vi "Programming Mode.vi"(8 "error in (no error)":errorcluster, 11 "serverName In":string="10.0.18.244") -> (0 "error out":errorcluster, 1 "Programming Mode Out":T1[](array[typedef]), 2 "Cancelled":bool, 3 "serverName Out":string="10.0.18.244")   [LabVIEW 2019, in "SEECD System Explorer.lvlib"]
doc: "This VI detects whether or not target local chassis supports \"Slot Programming Mode\" property.\nIf the case, populated slots have current value for the property displayed and user can change property.\nIf not the case, front-panel is not opened."
uses:
  SEECD System Explorer.lvlib
  Type Defs/Slot - Configuration.ctl
  Type Defs/Slot Programming Mode.ctl
  <vilib>/nisyscfg/Close (Resources).vi
  <vilib>/nisyscfg/Close (Filter).vi
  <vilib>/nisyscfg/Close (System).vi
  <vilib>/nisyscfg/nisyscfg.lvlib
panel:
  in  "Slot 7":T2 caption="Slot"
  in  "Slot 6":T2 caption="Slot"
  in  "Slot 5":T2 caption="Slot"
  in  "Slot 4":T2 caption="Slot"
  in  "Slot 3":T2 caption="Slot"
  in  "Slot 2":T2 caption="Slot"
  in  "Slot 1":T2 caption="Slot"
  in  "Slot 0":T2 caption="Slot"
  in  "User Name":string
  in  "Password":string
  in  "Set all modules to \"Scan Engine\" mode":bool
  in  "Cancel":bool
  in  "OK":bool
  # "Select a programming mode for detected modules and click \"OK\" button."
  # "New\nProgramming Mode"
  # "Current\nProgramming Mode"
  # "Module Name"
  # "Modules Name"
  # "Slot"
  # "Programming Mode"
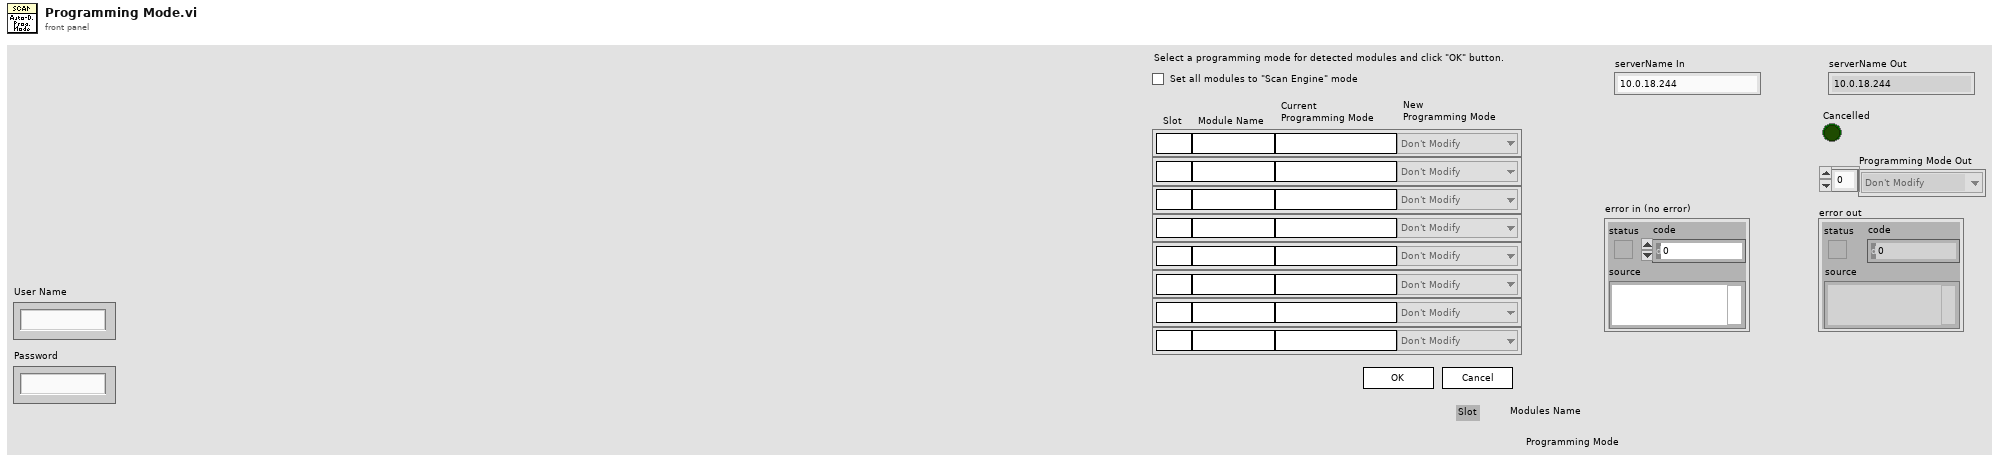
[diagram p1: front panel]
types:
  T1 = typedef "SEECD System Explorer.lvlib/Slot Programming Mode.ctl" = enum16{"Don't Modify", "Scan Engine", "LabVIEW FPGA", "NI-DAQmx"}
  T2 = typedef "SEECD System Explorer.lvlib/Slot - Configuration.ctl" = cluster{"Slot":string, "Module Name":string, "Current Prog Mode":string, "New Prog Mode":T1}
  T3 = enum32{"Invalid", "Standard", "Closed", "Hidden", "Minimized", "Maximized"}
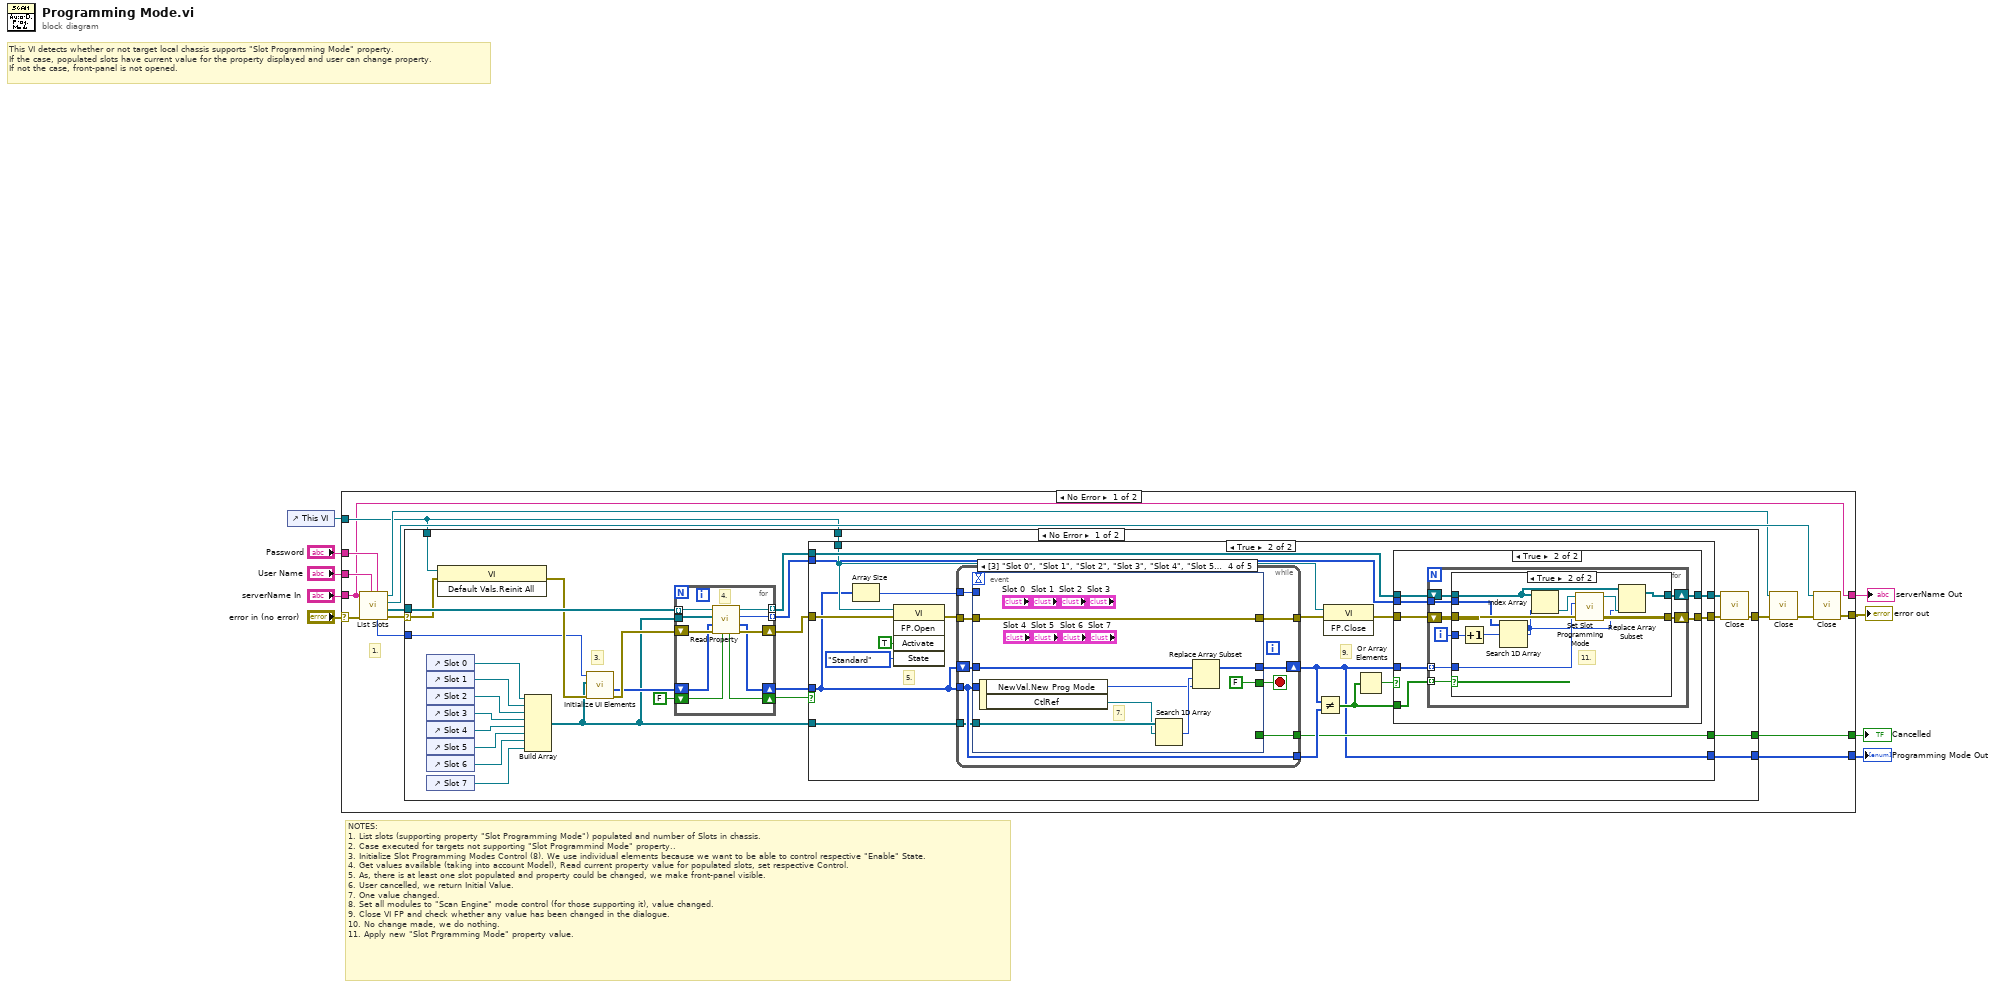
[diagram p0: block diagram]
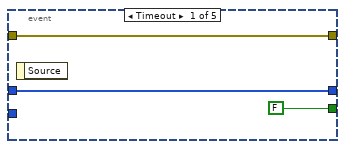
[diagram p3: hidden frame]
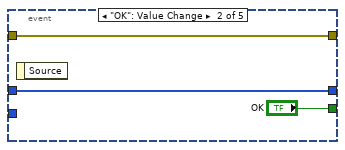
[diagram p4: hidden frame]
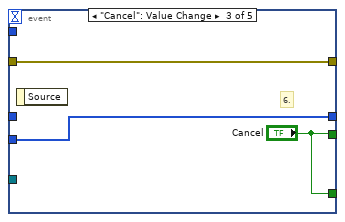
[diagram p5: hidden frame]
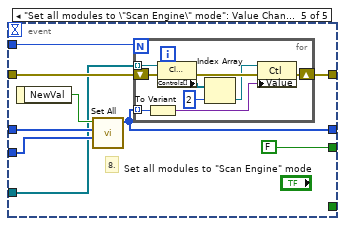
[diagram p6: hidden frame]
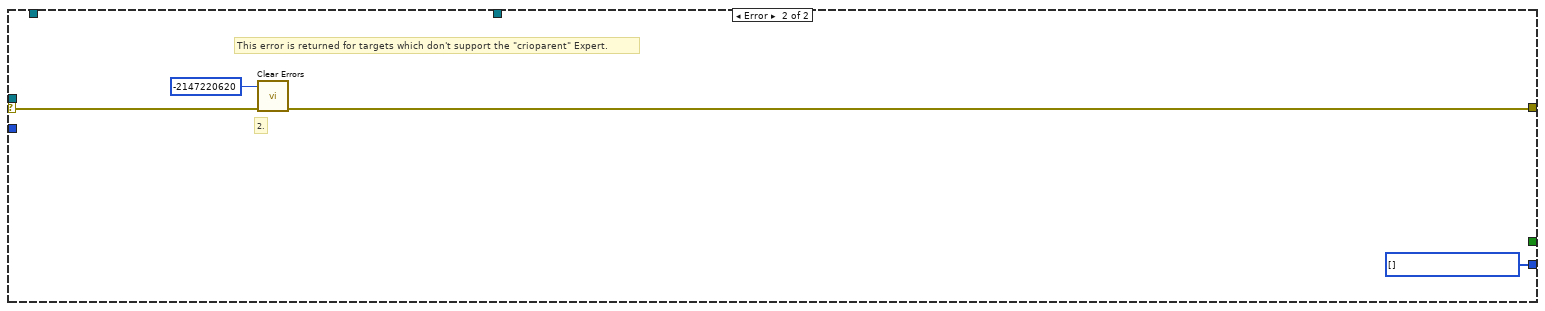
[diagram p9: hidden frame]
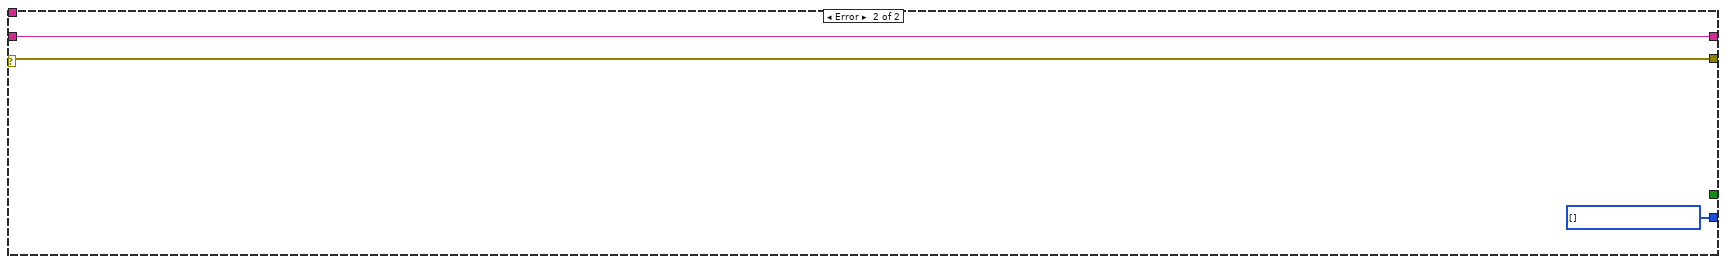
[diagram p10: hidden frame]
diagram:
  # "NOTES:\n1. List slots (supporting property \"Slot Programming Mode\") populated and number of Slots in chassis.\n2. Case executed for targets not supporting \"Slot Programmind Mode\" property..\n3. Initialize Slot Programming Modes Control (8). We use individual elements because we want to be able to control respective \"Enable\" State.\n4. Get values available (taking into account Model), Read current property value for populated slots, set respective Control.\n5. As, there is at least one slot populated and property could be changed, we make front-panel visible.\n6. User cancelled, we return Initial Value.\n7. One value changed.\n8. Set all modules to \"Scan Engine\" mode control (for those supporting it), value changed.\n9. Close VI FP and check whether any value has been changed in the dialogue.\n10. No change made, we do nothing.\n11. Apply new \"Slot Prgramming Mode\" property value."
  # "This VI detects whether or not target local chassis supports \"Slot Programming Mode\" property.\nIf the case, populated slots have current value for the property displayed and user can change property.\nIf not the case, front-panel is not opened."
  n1 = control-ref of="This VI"() -> (w4:refnum<vi>)
  n2 = case shown="No Error" "error in (no error)" {
    selector: "error in (no error)" -> [w23 w165]
    tunnel: "serverName In" -> [w13 w164]
    tunnel: "User Name" -> [w15 _]
    tunnel: "Password" -> [w14 _]
    tunnel: [w24 w165] -> w5
    tunnel: w4 -> [w16 _]
    tunnel: [w13 w164] -> w3
    tunnel: [w11 _] -> w2
    tunnel: [w10 w163] -> w1
    frame No Error {
      # "1."
      n3 = call "List Slots.vi"("Password"=w14, "User Name"=w15, "error in (no error)"=w23, "serverName In"=w13) -> ("error out"=w18:errorcluster, "Resources out"=w22:refnum<k20>[], "Session out"=w21:refnum<k21>, "Refnum out"=w17:refnum<k20>, "NumSlots"=w12:i32)  [unwired: 3 in]
      n4 = case shown="No Error" w18 {
        selector: w18 -> [w42 w162]
        tunnel: w22 -> [w52 _]
        tunnel: [w48 w160] -> w19
        tunnel: w16 -> [w47 _]
        tunnel: w16 -> [w43 _]
        tunnel: w12 -> [w29 _]
        tunnel: [w26 _] -> w11
        tunnel: [w25 w159] -> w10
        frame No Error {
          # "3."
          n5 = control-ref of="Slot 0"() -> (w34:refnum<vi>)
          n6 = control-ref of="Slot 1"() -> (w35:refnum<vi>)
          n7 = control-ref of="Slot 2"() -> (w36:refnum<vi>)
          n8 = control-ref of="Slot 3"() -> (w37:refnum<vi>)
          n9 = control-ref of="Slot 4"() -> (w38:refnum<vi>)
          n10 = control-ref of="Slot 5"() -> (w39:refnum<vi>)
          n11 = control-ref of="Slot 6"() -> (w40:refnum<vi>)
          n12 = control-ref of="Slot 7"() -> (w41:refnum<vi>)
          n13 = invoke class="VI" method="Default Vals.Reinit All"(reference=w43, error in=w42) -> (error out=w33:errorcluster)  [unwired: 1 in, 2 out]
          n14 = Build Array(w34, w35, w36, w37, w38, w39, w40, w41) -> (w27:refnum<vi>[])
          n15 = call "Initialize UI Elements.vi"("error in"=w33, "References"=w27, "NumSlots"=w29) -> ("error out"=w32:errorcluster, "Programming Mode Out"=w28:T1[])  [unwired: 7 in]
          n16 = for {
            tunnel: w52 -> [w154] mode=indexing
            shift-right: [w158] -> w49
            shift-left: w32 -> [w157]
            tunnel: [w153] -> w46 mode=indexing
            shift-right: [w150] -> w50
            shift-left: FALSE -> [w156]
            tunnel: w27 -> [w149]
            shift-right: [w151] -> w31
            shift-left: w28 -> [w155]
            tunnel: [w152] -> w30 mode=indexing
            # "4."
            n17 = call "Read Property.vi"("Initialized in"=w156, "error in (no error)"=w157, "Programming Mode In"=w155, "References"=w149, "Refnum in"=w154) -> ("error out"=w158:errorcluster, "Programming Mode Out"=w151:T1[], "Slot"=w152:i32, "Refnum out"=w153:refnum<k20>, "Initialized Out"=w150:bool)  [unwired: 2 in]
          }
          n18 = case shown="True" w50 {
            tunnel: w49 -> [w55 w62]
            tunnel: [w55 w65] -> w44
            tunnel: w31 -> [w53 w60]
            tunnel: w47 -> [_ w63]
            tunnel: w46 -> [w54 w69]
            tunnel: [w54 w64] -> w45
            tunnel: w27 -> [_ w61]
            tunnel: w30 -> [_ w58]
            tunnel: [_ w57] -> w26
            tunnel: [w53 w56] -> w25
            frame False {
            }
            frame True {
              # "9."
              # "5."
              n19 = Array Size(array=w60) -> (size(s)=w59:i32)
              n20 = invoke class="VI" method="FP.Open"(reference=w63, error in=w62, "Activate"=TRUE ("Activate?"), "State"=T3."Standard") -> (error out=w71:errorcluster)  [unwired: 1 in, 4 out]
              n21 = while {
                tunnel: w71 -> [w83]
                tunnel: w60 -> [w80]
                tunnel: [w80] -> w74
                tunnel: [w79] -> w70
                shift-right: [w81] -> w56
                shift-left: w60 -> [w78]
                tunnel: w61 -> [w77]
                tunnel: w59 -> [w76]
                tunnel: [w75] -> w57
                stop <- w82 stop-if-true
                n22 = event shown="[3] \"Slot 0\", \"Slot 1\", \"Slot 2\", \"Slot 3\", \"Slot 4\", \"Slot 5\", \"Slot 6\", \"Slot 7\": Value Change" {
                  selector: _ -> [_ _ _ _ _]
                  dyn-events: _ -> [_ _ _ _ _]
                  timeout: _ -> [_ _ _ _ _]
                  tunnel: w83 -> [w86 w88 w91 w99 w105]
                  tunnel: [FALSE ("Cancel") "OK" "Cancel" FALSE ("Cancel") FALSE ("Cancel")] -> w82
                  tunnel: [w85 w87 w92 w97 w103] -> w81
                  tunnel: w80 -> [_ _ w92 _ w104]
                  tunnel: [w86 w88 w91 w99 w106] -> w79
                  tunnel: w78 -> [w85 w87 _ w98 w107]
                  tunnel: w77 -> [_ _ _ w96 w102]
                  tunnel: w76 -> [_ _ _ _ w101]
                  tunnel: [_ _ "Cancel" _ _] -> w75
                  event Timeout {
                    n23 = event-data() -> ()  [unwired: 1 in, 1 out]
                  }
                  event "OK": Value Change {
                    n24 = event-data() -> ()  [unwired: 1 in, 1 out]
                  }
                  event "Cancel": Value Change {
                    # "6."
                    n25 = event-data() -> ()  [unwired: 1 in, 1 out]
                  }
                  event Value Change {
                    # "7."
                    n26 = event-data() -> ("NewVal.New Prog Mode"=w93:T1, "CtlRef"=w94:refnum<vi>)  [unwired: 1 in]
                    n27 = Search 1D Array(1D array=w96, element=w94) -> (index of element=w95:i32)  [unwired: 1 in]
                    n28 = Replace Array Subset(array=w98, new element=w93, index=w95) -> (w97:T1[])
                  }
                  event "Set all modules to \"Scan Engine\" mode": Value Change {
                    # "8."
                    n29 = event-data() -> ("NewVal"=w108:bool)  [unwired: 1 in]
                    n30 = call "Set All.vi"("Init Value"=w104, "Previous Value"=w107, "Set ALL NewVal"=w108) -> ("Value Out"=w103:T1[])  [unwired: 8 in]
                    n31 = for {
                      N: w101 -> [_]
                      tunnel: w103 -> [w111] mode=indexing
                      shift-right: [w112] -> w106
                      shift-left: w105 -> [w118]
                      tunnel: w102 -> [w117] mode=indexing
                      n32 = To Variant(anything=w111) -> (Variant=w110:variant)
                      n33 = property class="Clust (strict)"(reference=w117, error in=w118) -> (error out=w114:errorcluster, "Controls[]"=w116:refnum<vi>[])  [unwired: 1 out]
                      n34 = Index Array(array=w116, index=2) -> (element=w113:refnum<vi>)
                      n35 = property class="Ctl"(reference=w113, error in=w114, "Value"=w110) -> (error out=w112:errorcluster)  [unwired: 1 out]
                    }
                  }
                }
              }
              n36 = Not Equal?(x=w56, y=w74) -> (x != y?=w66:bool[])
              n37 = invoke class="VI" method="FP.Close"(reference=w63, error in=w70) -> (error out=w68:errorcluster)  [unwired: 1 in, 2 out]
              n38 = Or Array Elements(Boolean array=w66) -> (logical OR=w67:bool)
              n39 = case shown="True" w67 {
                tunnel: w69 -> [w119 w127]
                tunnel: w68 -> [w120 w126]
                tunnel: w66 -> [_ w125]
                tunnel: w56 -> [_ w124]
                tunnel: [w120 w123] -> w65
                tunnel: [w119 w122] -> w64
                tunnel: w58 -> [_ w121]
                frame False {
                  # "10."
                }
                frame True {
                  n40 = for {
                    tunnel: w125 -> [w135] mode=indexing
                    tunnel: w124 -> [w134] mode=indexing
                    shift-right: [w131] -> w123
                    shift-left: w126 -> [w133]
                    tunnel: w121 -> [w128]
                    shift-right: [w130] -> w122
                    shift-left: w127 -> [w132]
                    i -> [w129]
                    n41 = case shown="True" w135 {
                      tunnel: w134 -> [_ w146]
                      tunnel: w133 -> [w137 w148]
                      tunnel: w132 -> [w136 w140]
                      tunnel: [w137 w147] -> w131
                      tunnel: [w136 w138] -> w130
                      tunnel: w129 -> [_ w144]
                      tunnel: w128 -> [_ w145]
                      frame False {
                      }
                      frame True {
                        # "11."
                        n42 = Increment(x=w144) -> (x+1=w143:i32)
                        n43 = Search 1D Array(1D array=w145, element=w143) -> (index of element=w139:i32)  [unwired: 1 in]
                        n44 = Index Array(array=w140, index=w139) -> (element=w142:refnum<k20>)
                        n45 = call "Set Slot Programming Mode.vi"("error in (no error)"=w148, "Slot Programming Mode"=w146, "Refnum in"=w142) -> ("error out"=w147:errorcluster, "Refnum out"=w141:refnum<k20>)  [unwired: 7 in]
                        n46 = Replace Array Subset(array=w140, new element=w141, index=w139) -> (w138:refnum<k20>[])
                      }
                    }
                  }
                }
              }
            }
          }
          n47 = call-poly <vilib>:"Close.vi"("error in (no error)"=w44, "Resources in"=w45) -> ("error out"=w48:errorcluster)  [unwired: 9 in]
        }
        frame Error {
          w159 = T1[] [] items=["Don't Modify", "Scan Engine", "LabVIEW FPGA", "NI-DAQmx"] ("Programming Mode Out")
          # "2."
          # "This error is returned for targets which don't support the \"crioparent\" Expert."
          n48 = call <vilib>:"Clear Errors.vi"("error in (no error)"=w162, "specific error code to clear (0: all)"=-2147220620) -> ("error out"=w160:errorcluster)  [unwired: 4 in, 1 out]
        }
      }
      n49 = call-poly <vilib>:"Close.vi"("error in (no error)"=w19, "Filter in"=w17) -> ("error out"=w20:errorcluster)  [unwired: 9 in]
      n50 = call-poly <vilib>:"Close.vi"("error in (no error)"=w20, "Session in"=w21) -> ("error out"=w24:errorcluster)  [unwired: 9 in]
    }
    frame Error {
      w163 = T1[] [] items=["Don't Modify", "Scan Engine", "LabVIEW FPGA", "NI-DAQmx"] ("Programming Mode Out")
    }
  }
  "error out" <- w5
  "serverName Out" <- w3
  "Cancelled" <- w2
  "Programming Mode Out" <- w1
